vi "RIO_Terminal.vi"() -> ()   [LabVIEW 2012]
panel:
  out "Tasks":i32(listbox)
  in  "Load exe":bool
  in  "Get exe":bool
  out "startup there?":bool
  in  "Upload Latest VM":bool
  out "ini file":string
  out "old autolaunch state":bool
  in  "user":string
  in  "password":string
  in  "address":string="169.254.66.100"
  out "Good?":bool[](array[boolean])
  out "Done":string
  in  "Directories":enum32{"Main", "startup"}(tab)
  out "Main Directory":string
  out "startup dir":string
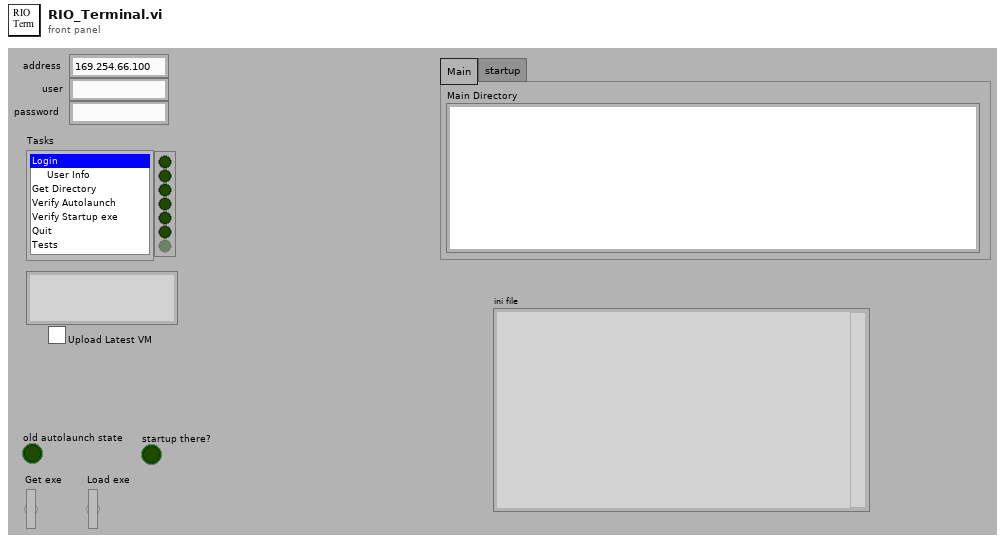
[diagram p1: front panel]
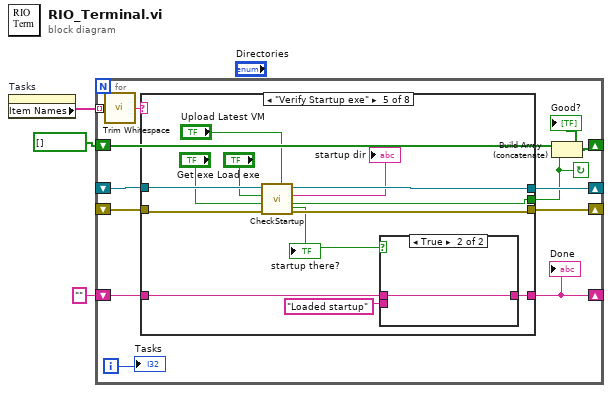
[diagram p0: block diagram]
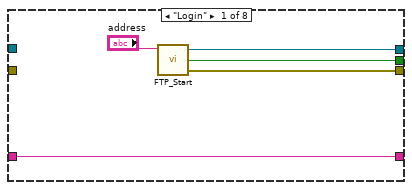
[diagram p2: hidden frame]
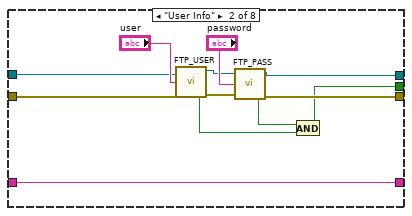
[diagram p3: hidden frame]
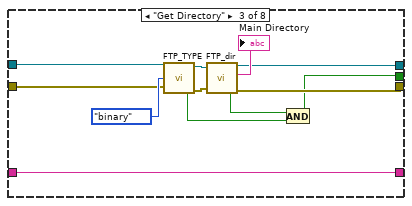
[diagram p4: hidden frame]
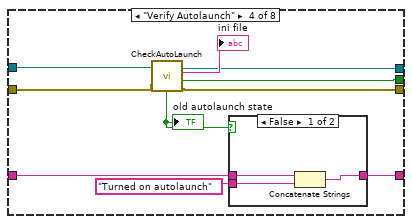
[diagram p5: hidden frame]
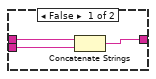
[diagram p7: hidden frame]
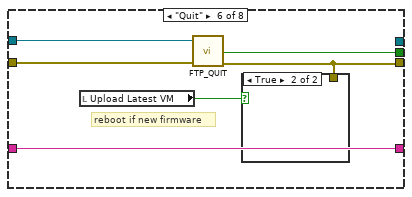
[diagram p8: hidden frame]
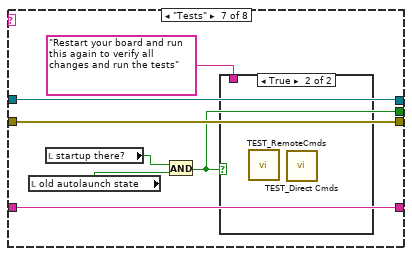
[diagram p10: hidden frame]
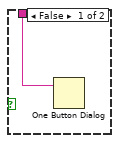
[diagram p11: hidden frame]
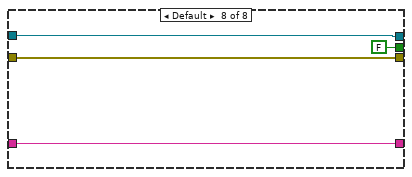
[diagram p12: hidden frame]
diagram:
  n1 = property on="Tasks" class="LstBox (strict)"() -> ("Item Names"=w3:string[])  [unwired: 2 in, 2 out]
  n2 = for {
    tunnel: w3 -> [w14] mode=indexing
    shift-right: [w12] -> _
    shift-left: _ -> [w11]
    shift-right: [w13] -> _
    shift-left: _ -> [w10]
    shift-right: [w8] -> _
    shift-left: bool[] [] -> [w9]
    shift-right: [w4] -> _
    shift-left: "" -> [w5]
    i -> [w15]
    stop <- w7 continue-if-true
    n3 = call <vilib>:"Trim Whitespace.vi"("string"=w14) -> ("trimmed string"=w6:string)  [unwired: 1 in]
    n4 = case shown="\"Verify Startup exe\"" w6 {
      tunnel: [w19 w26 w38 w52 w69 w77 w87 w92] -> w13
      tunnel: [w18 w25 w37 w51 w70 _ w88 w93] -> w12
      tunnel: w11 -> [_ w27 w40 w53 w71 w81 w88 w93]
      tunnel: w10 -> [_ w28 w39 w50 w68 w80 w87 w92]
      tunnel: [w17 w22 w34 w49 w65 w79 w84 FALSE ("Good Reply?")] -> w7
      tunnel: w5 -> [w16 w21 w33 w47 w62 w78 w86 w90]
      tunnel: [w16 w21 w33 w45 w63 w78 w86 w90] -> w4
      frame "Login" {
        n5 = call <userlib>:"FTP_Start.vi"("address"="address") -> ("connection ID"=w18:refnum<k5>, "Good Reply?"=w17:bool, "error out"=w19:errorcluster)  [unwired: 4 in]
      }
      frame "User Info" {
        n6 = call <userlib>:"FTP_USER.vi"("connection ID"=w27, "user"="user", "error out"=w28) -> ("connection ID out"=w29:refnum<k5>, "Good Reply?"=w24:bool, "error out 2"=w30:errorcluster)  [unwired: 1 out]
        n7 = call <userlib>:"FTP_PASS.vi"("connection ID"=w29, "password"="password", "error in"=w30) -> ("connection ID out"=w25:refnum<k5>, "Good Reply?"=w23:bool, "error out"=w26:errorcluster)  [unwired: 1 out]
        n8 = And(x=w23, y=w24) -> (x .and. y?=w22:bool)
      }
      frame "Get Directory" {
        n9 = call <userlib>:"FTP_TYPE.vi"("connection ID"=w40, "type (query)"=enum16{"(query)", "ASCII", "binary"}."binary", "error in"=w39) -> ("connection ID out"=w41:refnum<k5>, "Good Reply?"=w36:bool, "error out"=w42:errorcluster)  [unwired: 1 out]
        n10 = call <userlib>:"FTP_dir.vi"("connection ID"=w41, "error in"=w42) -> ("connection ID out"=w37:refnum<k5>, "reply string"=→"Main Directory":string, "Good Reply?"=w35:bool, "error out"=w38:errorcluster)  [unwired: 1 out]
        n11 = And(x=w35, y=w36) -> (x .and. y?=w34:bool)
      }
      frame "Verify Autolaunch" {
        n12 = call <userlib>:"CheckAutoLaunch.vi"("error in"=w50, "connection ID in"=w53) -> ("AutoLaunch?"=w48:bool, "error out"=w52:errorcluster, "Good Reply?"=w49:bool, "ini file"=→"ini file":string, "connection ID out"=w51:refnum<k5>)  [unwired: 1 in]
        "old autolaunch state" <- w48
        n13 = case shown="False" w48 {
          tunnel: w47 -> [w57 w58]
          tunnel: "Turned on autolaunch" ("string") -> [w56 _]
          tunnel: [w55 w58] -> w45
          frame False {
            n14 = Concatenate Strings(w57, w56) -> (w55:string)
          }
          frame True {
          }
        }
      }
      frame "Verify Startup exe" {
        n15 = call <userlib>:"CheckStartup.vi"("error in"=w68, "Get exe"="Get exe", "Load exe"="Load exe", "connection ID in"=w71, "Load latest"="Upload Latest VM") -> ("startup there?"=w61:bool, "error out"=w69:errorcluster, "Good Reply?"=w65:bool, "startup dir"=→"startup dir":string, "connection ID out"=w70:refnum<k5>)
        "startup there?" <- w61
        n16 = case shown="True" w61 {
          tunnel: w62 -> [w74 w75]
          tunnel: "Loaded startup" ("string") -> [w73 _]
          tunnel: [w72 w75] -> w63
          frame False {
            n17 = Concatenate Strings(w74, w73) -> (w72:string)
          }
          frame True {
          }
        }
      }
      frame "Quit" {
        # "reboot if new firmware"
        n18 = local read "Upload Latest VM"() -> (w76:bool)
        n19 = call <userlib>:"FTP_QUIT.vi"("connection ID"=w81, "error in"=w80) -> ("Good Reply?"=w79:bool, "error out"=w77:errorcluster)  [unwired: 2 out]
        n20 = case shown="True" w76 {
          tunnel: w77 -> [_ _]
          frame False {
          }
          frame True {
          }
        }
      }
      frame "Tests" {
        n21 = local read "old autolaunch state"() -> (w85:bool)
        n22 = local read "startup there?"() -> (w82:bool)
        n23 = And(x=w82, y=w85) -> (x .and. y?=w84:bool)
        n24 = case shown="True" w84 {
          tunnel: "Restart your board and run this again to verify all changes and run the tests" -> [w89 _]
          frame False {
            n25 = One Button Dialog(message=w89) -> ()  [unwired: 1 in, 1 out]
          }
          frame True {
            n26 = call <userlib>:"TEST_RemoteCmds.vi"() -> ()  [unwired: 12 in]
            n27 = call <userlib>:"TEST_Direct Cmds.vi"() -> ()  [unwired: 12 in]
          }
        }
      }
      frame Default {
      }
    }
    "Done" <- w4
    n28 = Build Array (concatenate)(w9, w7) -> (w8:bool[])
    "Good?" <- w8
    "Tasks" <- w15
  }
